vi "ZE_Recorder_ConfigFGV.vi"(7 "XML cluster in":T1={"SettingsCluster"={"Header Cluster"={"Project"="", "Operator ID"="", "Description"="(replace) Measurement Description (replace):"}, "Sampling Rate [Hz]"=100.0, "Channel Array"=[], "File Cluster"={"File Postfix"="", "Folder"=path "C:/Users/pats/Documents/LabVIEW Data", "File Type"=enum."CSV"}}} caption="output cluster" {"SettingsCluster"."Channel Array"."Terminal" items=["Default"=-1, "RSE"=10083, "NRSE"=10078, "Differential"=10106, "Pseudodifferential"=12529]; "SettingsCluster"."Sampling Rate [Hz]" min=0.001 max=1000000.0 step=0.1}, 8 "error in":errorcluster={"status"=TRUE, "code"=1025, "source"="Property Node in ZE_Recorder_Initalize.vi"}, 9 "Action":T9=enum."Open File", 10 "Application in":refnum<vi>) -> (0 "error out":errorcluster, 5 "XML cluster out":T1={"SettingsCluster"={"Header Cluster"={"Project"="", "Operator ID"="", "Description"="(replace) Measurement Description (replace):"}, "Sampling Rate [Hz]"=100.0, "Channel Array"=[], "File Cluster"={"File Postfix"="", "Folder"=path "C:/Users/pats/Documents/LabVIEW Data", "File Type"=enum."CSV"}}} caption="output cluster" {"SettingsCluster"."Channel Array"."Terminal" items=["Default"=-1, "RSE"=10083, "NRSE"=10078, "Differential"=10106, "Pseudodifferential"=12529]; "SettingsCluster"."Sampling Rate [Hz]" min=0.001 max=1000000.0 step=0.1})   [LabVIEW 2025, in "ZE_Recorder.lvlib"]
doc: "ZE_Recorder_ConfigFGV.vi\n----------------------------------------------\nThe VI serves as an FGV containing the path to the parameter config XML as well as providing the functions for reading from and saving to the XML file.\n\nInputs:\n---------------------\n- Action : EnumU16; \n- Application in : Refnum; \n- Data cluster : Cluster; \n\nOutputs:\n---------------------\n- Data cluster out : Cluster; \n\n----------------------------------------------\n02.06.2016\nZühlke Engineering AG\nCH-8952 Schlieren\nwww.zuehlke.com"
uses:
  ZE_Recorder.lvlib
  XmlFileAction.ctl
  ZE_Recorder_XMLCluster.ctl
  ZE_Recorder_Settings.ctl
  ZE_Recorder_Header.ctl
  ZE_Recorder_ChannelCluster.ctl
  ChannelCluster.ctl
  ZE_Recorder_Units.ctl
  Temperature.ctl
  ZE_Recorder_FileCluster.ctl
  LVLIBP/ZE_APP_Application.lvlibp/ZE_APP_DefaultAppPaths_State.ctl
  <vilib>/Utility/xml.llb/Write to XML File(string).vi
  <vilib>/Utility/xml.llb/Read From XML File(string).vi
  LVLIBP/ZE_APP_Application.lvlibp
panel:
  # "Project Info"
  # "Channel Settings"
  # "Result File Settings"
  # "."
  # "Project Info"
  # "Channel Settings"
  # "Result File Settings"
  # "."
  # "Connector Pane"
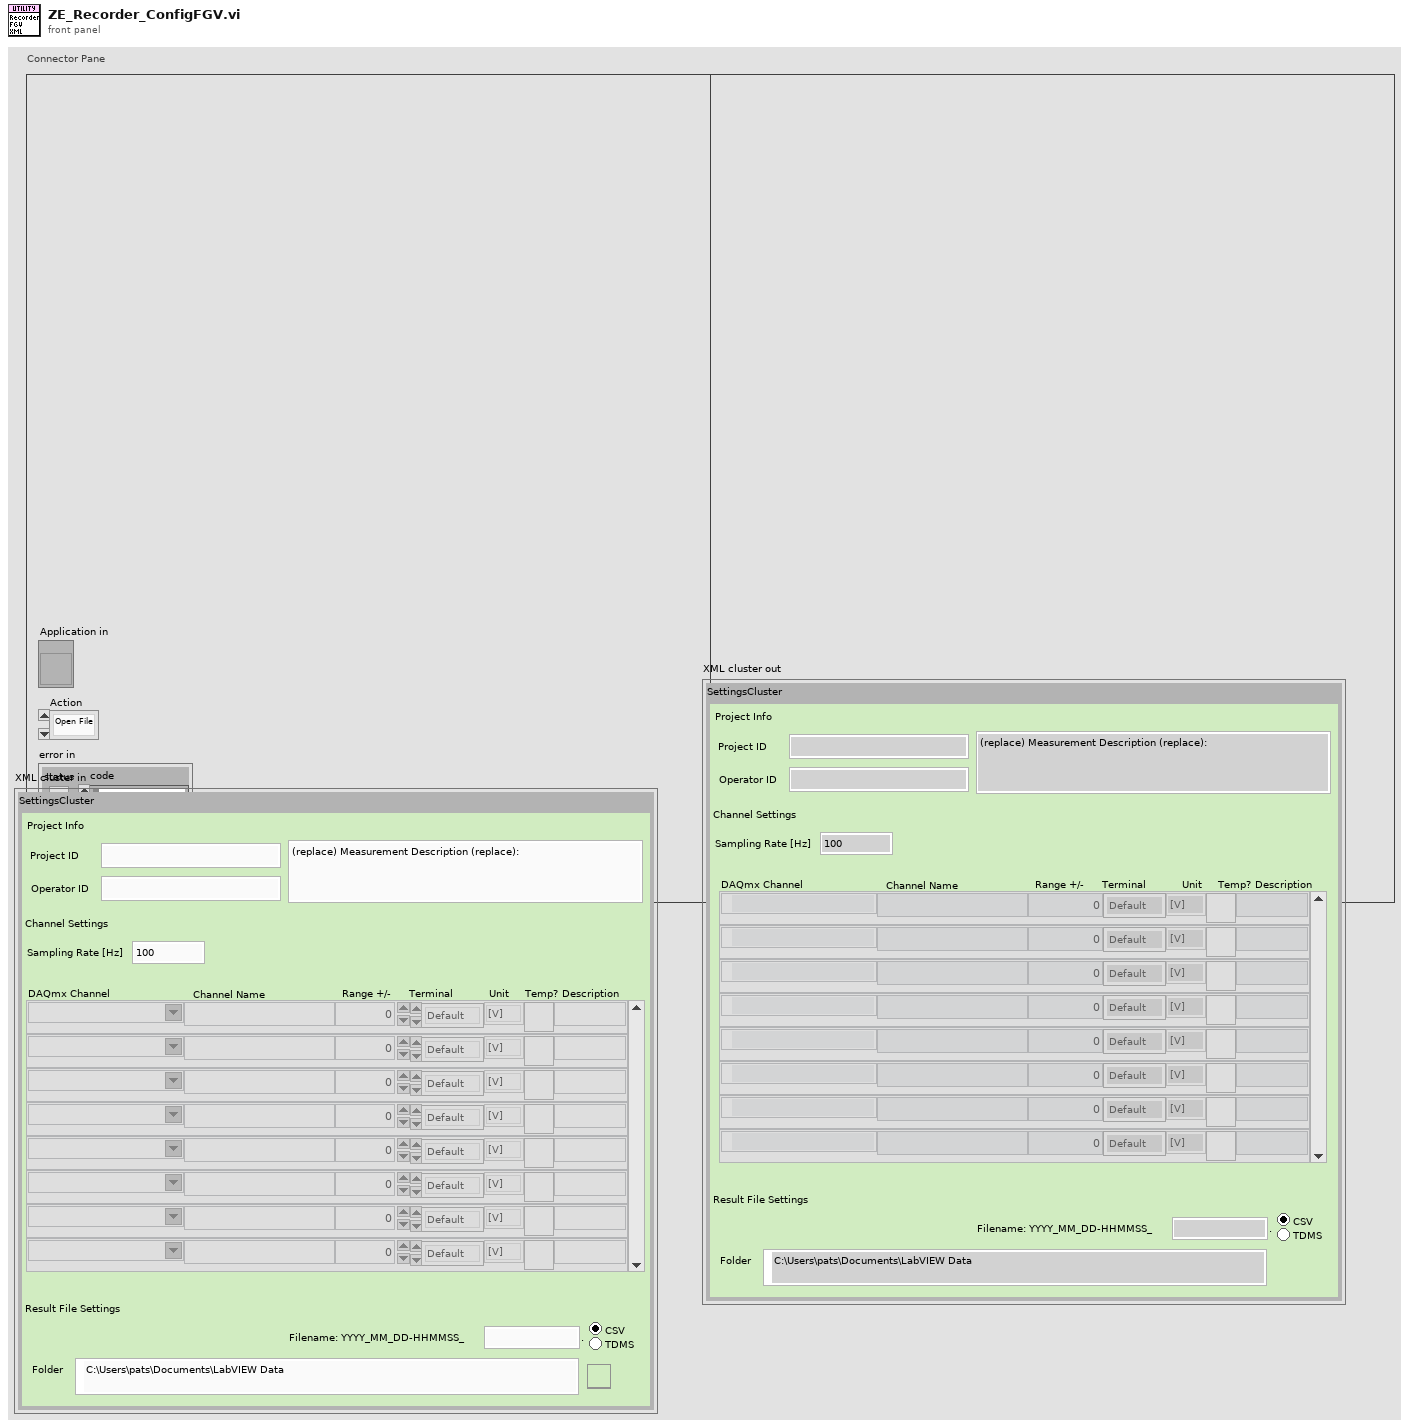
[diagram p1: front panel]
types:
  T1 = typedef "ZE_Recorder.lvlib/ZE_Recorder_XMLCluster.ctl" = cluster{"SettingsCluster":T2}
  T2 = typedef "ZE_Recorder.lvlib/ZE_Recorder_Settings.ctl" = cluster{"Header Cluster":T3, "Sampling Rate [Hz]":dbl, "Channel Array":T4, "File Cluster":T8}
  T3 = typedef "ZE_Recorder.lvlib/ZE_Recorder_Header.ctl" = cluster{"Project":string, "Operator ID":string, "Description":string}
  T4 = typedef "ZE_Recorder.lvlib/ZE_Recorder_ChannelCluster.ctl" = T5[]
  T5 = typedef "ZE_Recorder.lvlib/ChannelCluster.ctl" = cluster{"physical channel":tag, "channel name":string, "Range":dbl, "Terminal":i32, "Unit":T6, "isTemp":T7, "Description":string}
  T6 = typedef "ZE_Recorder.lvlib/ZE_Recorder_Units.ctl" = enum16{"[V]", "[A]", "[F]", "[H]", "[°C]", "[ml/s]", "[m/s]", "[bar]", "[%]", "[N]", "[?]"}
  T7 = typedef "ZE_Recorder.lvlib/Temperature.ctl" = bool
  T8 = typedef "ZE_Recorder.lvlib/ZE_Recorder_FileCluster.ctl" = cluster{"File Postfix":string, "Folder":path, "File Type":enum32{"CSV", "TDMS"}}
  T9 = typedef "ZE_Recorder.lvlib/XmlFileAction.ctl" = enum16{"Write and Close File", "WriteFileAs", "Open File", "OpenFileWithDialog"}
  T10 = typedef "ZE_APP_Application.lvlibp/ZE_APP_DefaultAppPaths_State.ctl" = enum16{"Init", "Read", "Write"}
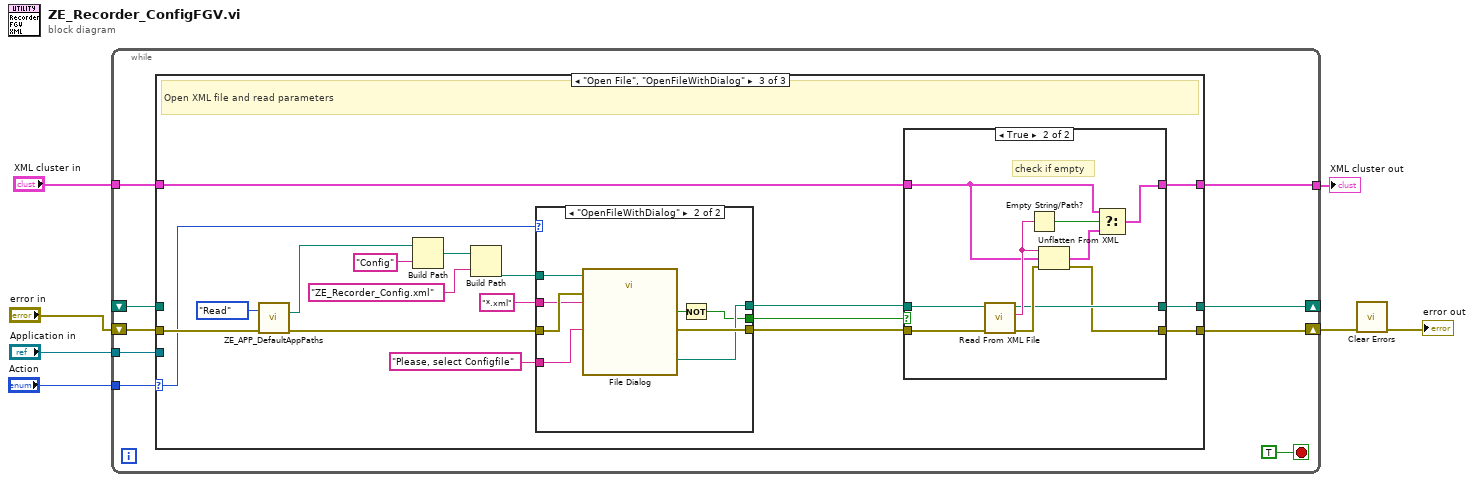
[diagram p0: block diagram]
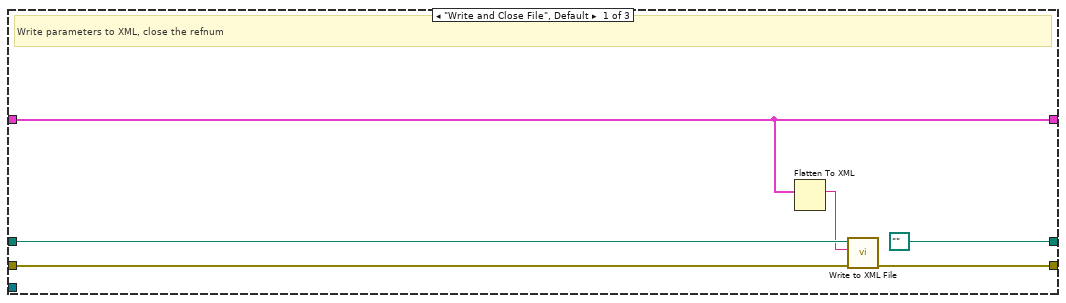
[diagram p2: hidden frame]
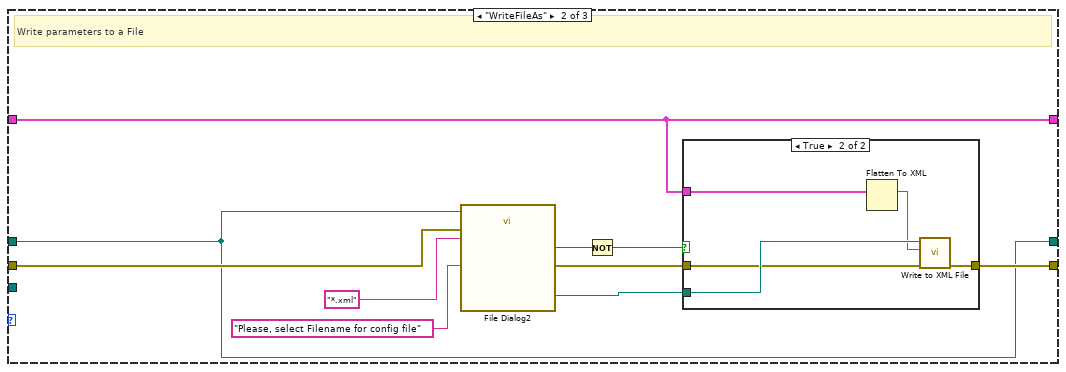
[diagram p3: hidden frame]
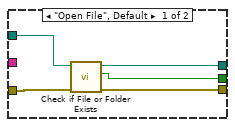
[diagram p5: hidden frame]
diagram:
  n1 = while {
    tunnel: "Application in" -> [w16]
    shift-right: [w14] -> _
    shift-left: _ -> [w12]
    tunnel: "Action" -> [w13]
    tunnel: "XML cluster in" -> [w11]
    shift-right: [w10] -> w3
    shift-left: "error in" -> [w9]
    tunnel: [w8] -> w1
    stop <- TRUE stop-if-true
    n2 = case shown="\"Open File\", \"OpenFileWithDialog\"" w13 {
      selector: w13 -> [_ _ w44]
      tunnel: w16 -> [_ _ _]
      tunnel: [path "" ("appended path") w27 w55] -> w14
      tunnel: w12 -> [w22 w27 _]
      tunnel: w11 -> [w17 w23 w54]
      tunnel: w9 -> [w20 w28 w56]
      tunnel: [w19 w32 w53] -> w10
      tunnel: [w17 w23 w45] -> w8
      frame "Write and Close File", Default {
        # "Write parameters to XML, close the refnum"
        n3 = Flatten To XML(6:w17) -> (2:w21:string)
        n4 = call-poly <vilib>:"Write to XML File.vi"("error in (no error)"=w20, "XML Input"=w21, "XML File Path"=w22) -> ("error out"=w19:errorcluster)  [unwired: 6 in, 2 out]
      }
      frame "WriteFileAs" {
        # "Write parameters to a File"
        n5 = call "File Dialog2"("start path"=w27, "prompt"="Please, select Filename for config file" ("pattern (all files)"), "error in"=w28, "pattern (all files)"="*.xml") -> ("selected path"=w25:path, "cancelled"=w24:bool, "error out"=w29:errorcluster)  [unwired: 8 in, 1 out]
        n6 = Not(x=w24) -> (.not. x?=w26:bool)
        n7 = case shown="True" w26 {
          tunnel: w23 -> [_ w34]
          tunnel: w25 -> [_ w38]
          tunnel: w29 -> [w33 w36]
          tunnel: [w33 w35] -> w32
          frame False {
          }
          frame True {
            n8 = Flatten To XML(6:w34) -> (2:w37:string)
            n9 = call-poly <vilib>:"Write to XML File.vi"("error in (no error)"=w36, "XML Input"=w37, "XML File Path"=w38) -> ("error out"=w35:errorcluster)  [unwired: 6 in, 2 out]
          }
        }
      }
      frame "Open File", "OpenFileWithDialog" {
        # "Open XML file and read parameters"
        n10 = call "ZE_APP_DefaultAppPaths.vi"("State"=ZE_APP_DefaultAppPaths_State."Read", "ErrorIn"=w56) -> ("AppDataPath"=w40:path, "ErrorOut"=w52:errorcluster)  [unwired: 10 in, 2 out]
        n11 = Build Path(base path=w40, name or relative path="Config") -> (appended path=w39:path)
        n12 = Build Path(base path=w39, name or relative path="ZE_Recorder_Config.xml") -> (appended path=w51:path)
        n13 = case shown="\"OpenFileWithDialog\"" w44 {
          tunnel: w52 -> [w61 w69]
          tunnel: [w60 w68] -> w47
          tunnel: w51 -> [w59 w67]
          tunnel: [w58 w66] -> w49
          tunnel: "*.xml" ("pattern (all files)") -> [_ w65]
          tunnel: [w57 w62] -> w48
          tunnel: "Please, select Configfile" ("pattern (all files)") -> [_ w64]
          frame "Open File", Default {
            n14 = call <vilib>:"Check if File or Folder Exists.vi"("error in (no error)"=w61, "path"=w59) -> ("error out"=w60:errorcluster, "file or folder exists?"=w57:bool, "dup path"=w58:path)  [unwired: 7 in]
          }
          frame "OpenFileWithDialog" {
            n15 = call "File Dialog"("start path"=w67, "prompt"=w64, "error in"=w69, "pattern (all files)"=w65) -> ("selected path"=w66:path, "cancelled"=w63:bool, "error out"=w68:errorcluster)  [unwired: 8 in, 1 out]
            n16 = Not(x=w63) -> (.not. x?=w62:bool)
          }
        }
        n17 = case shown="True" w48 {
          tunnel: w47 -> [w71 w82]
          tunnel: w49 -> [w72 w81]
          tunnel: [w72 w78] -> w55
          tunnel: w54 -> [w70 w73]
          tunnel: [w71 w77] -> w53
          tunnel: [w70 w74] -> w45
          frame False {
          }
          frame True {
            # "check if empty"
            n18 = call-poly <vilib>:"Read From XML File.vi"("error in (no error)"=w82, "XML File Path"=w81) -> ("error out"=w80:errorcluster, "XML Elements"=w79:string, "XML File Path(duplicate)"=w78:path)  [unwired: 7 in]
            n19 = Empty String/Path?(string/path=w79) -> (empty?=w76:bool)
            n20 = Unflatten From XML(xml string=w79, type=w73, error in (no error)=w80) -> (value=w75:T1, error out=w77:errorcluster)
            n21 = Select(t=w73, s=w76, f=w75) -> (s? t:f=w74:T1)
          }
        }
      }
    }
  }
  "XML cluster out" <- w1
  n22 = call <vilib>:"Clear Errors.vi"("error in (no error)"=w3) -> ("error out"=→"error out":errorcluster)  [unwired: 5 in, 1 out]
